vi "CalculateRotorBar.vi"(6 "Calculation Cache In":T2 {"speed initial conditions"."zoom FFT settings"."FFT settings"."window" items=["Rectangle"=0, "Hanning"=1, "Hamming"=2, "Blackman-Harris"=3, "Exact Blackman"=4, "Blackman"=5, "Flat Top"=6, "4 Term B-Harris "=7, "7 Term B-Harris"=8, "Low Sidelobe"=9, "Blackman Nuttall"=11, "Triangle"=30, "Bartlett-Hanning"=31, "Bohman"=32, "Parzen"=33, "Welch"=34, "Kaiser"=60, "Dolph-Chebyshev"=61, "Gaussian"=62]; "spectrum initial conditions"."zoom FFT settings"."FFT settings"."window" items=["Rectangle"=0, "Hanning"=1, "Hamming"=2, "Blackman-Harris"=3, "Exact Blackman"=4, "Blackman"=5, "Flat Top"=6, "4 Term B-Harris "=7, "7 Term B-Harris"=8, "Low Sidelobe"=9, "Blackman Nuttall"=11, "Triangle"=30, "Bartlett-Hanning"=31, "Bohman"=32, "Parzen"=33, "Welch"=34, "Kaiser"=60, "Dolph-Chebyshev"=61, "Gaussian"=62]}, 8 "error in (no error)":errorcluster, 9 "Map":T1, 10 "current waveform":waveform(dbl)[](array[waveform]), 11 "voltage waveform":waveform(dbl)[](array[waveform])) -> (0 "error out":errorcluster, 3 "max sideband magnitude [dB]":dbl, 4 "Calculation Cache Out":T2 {"speed initial conditions"."zoom FFT settings"."FFT settings"."window" items=["Rectangle"=0, "Hanning"=1, "Hamming"=2, "Blackman-Harris"=3, "Exact Blackman"=4, "Blackman"=5, "Flat Top"=6, "4 Term B-Harris "=7, "7 Term B-Harris"=8, "Low Sidelobe"=9, "Blackman Nuttall"=11, "Triangle"=30, "Bartlett-Hanning"=31, "Bohman"=32, "Parzen"=33, "Welch"=34, "Kaiser"=60, "Dolph-Chebyshev"=61, "Gaussian"=62]; "spectrum initial conditions"."zoom FFT settings"."FFT settings"."window" items=["Rectangle"=0, "Hanning"=1, "Hamming"=2, "Blackman-Harris"=3, "Exact Blackman"=4, "Blackman"=5, "Flat Top"=6, "4 Term B-Harris "=7, "7 Term B-Harris"=8, "Low Sidelobe"=9, "Blackman Nuttall"=11, "Triangle"=30, "Bartlett-Hanning"=31, "Bohman"=32, "Parzen"=33, "Welch"=34, "Kaiser"=60, "Dolph-Chebyshev"=61, "Gaussian"=62]})   [LabVIEW 2017, in "McsaAnalysisFunctions.lvlib"]
uses:
  <vilib>/addons/InsightCM/Utilities/Analysis/MCSA/McsaAnalysisFunctions.lvlib
  <vilib>/addons/InsightCM/Utilities/Analysis/MCSA/controls/McsaCalculationCache.ctl
  <vilib>/addons/Electrical Power/Motor Monitoring/subVIs/ep_Initial Conditions for MCSA Spectra.ctl
  <vilib>/addons/Electrical Power/Motor Monitoring/subVIs/ep_Demodulation Algorithm.ctl
  <vilib>/addons/Electrical Power/Motor Monitoring/subVIs/ep_Zoom FFT Settings.ctl
  <vilib>/addons/Electrical Power/Motor Monitoring/subVIs/ep_Initial Conditions for Speed Estimation.ctl
  <vilib>/addons/PointValueMap/controls/PointMap.ctl
  <vilib>/addons/Electrical Power/Motor Monitoring/subVIs/ep_Spectra Settings.ctl
  <vilib>/addons/Electrical Power/Motor Monitoring/MCSA Spectra (1 Motor with IC).vi
  <vilib>/addons/Electrical Power/Motor Monitoring/Broken Rotor Bar Harmonics (1 Motor).vi
  <vilib>/addons/Electrical Power/Motor Monitoring/NI_EP_Motor Monitoring.lvlib
  <vilib>/addons/PointValueMap/PointValueMap.lvlib
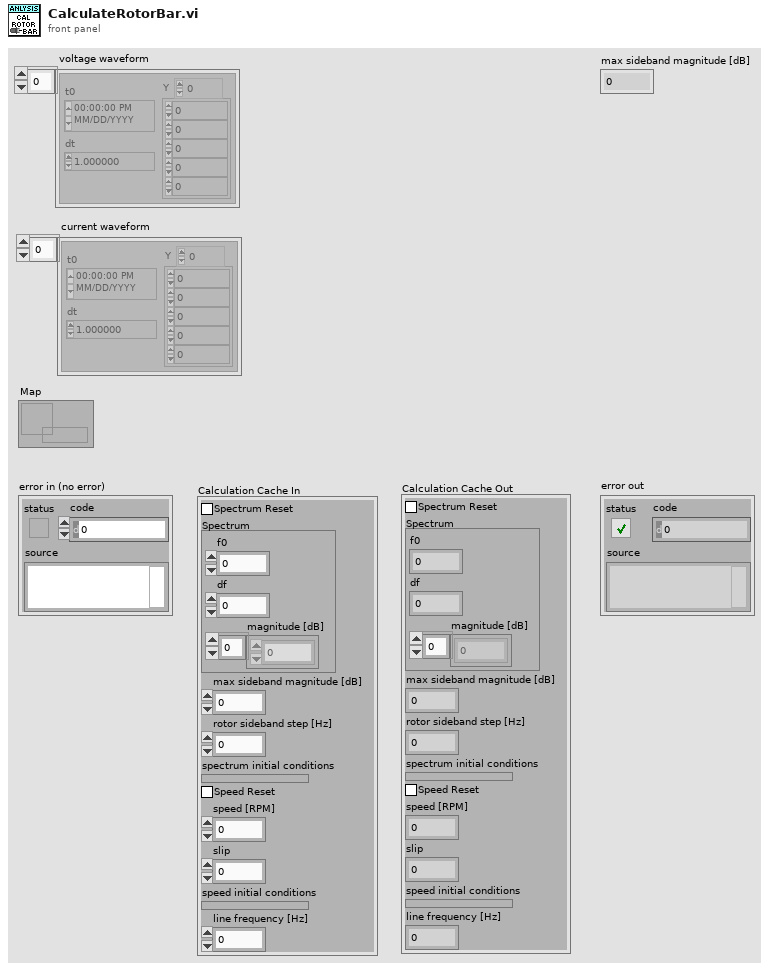
[diagram p1: front panel]
types:
  T1 = typedef "PointValueMap.lvlib/PointMap.ctl" = refnum<data-value>
  T2 = typedef "McsaAnalysisFunctions.lvlib/McsaCalculationCache.ctl" = cluster{"Spectrum Reset":bool, "Spectrum":cluster{"f0":dbl, "df":dbl, "magnitude [dB]":dbl[]}, "max sideband magnitude [dB]":dbl, "rotor sideband step [Hz]":dbl, "spectrum initial conditions":T3, "Speed Reset":bool, "speed [RPM]":dbl, "slip":dbl, "speed initial conditions":T6, "line frequency [Hz]":dbl}
  T3 = typedef "NI_EP_Motor Monitoring.lvlib/ep_Initial Conditions for MCSA Spectra.ctl" = cluster{"hilbert state":cluster{"delay conditions":dbl[], "filter conditions":dbl[]}, "zoom FFT state":cluster{"phase state":dbl, "zoom FFT state":cluster{"zoom settings state":cluster{"zoom":i32, "stop band attenuation":enum16{"84 dB", "96 dB", "120 dB"}, "alias protect in final transition":bool, "oversampling ratio":dbl}, "SML Decimation Filter (complex input) state":cluster{"decimation settings state":cluster{"M":i32, "stop band attenuation":enum16{"84 dB", "96 dB", "120 dB"}, "alias protect in transition band":bool, "oversampling ratio":dbl}, "counter for garbage samples state":i32, "sml_Parameter Setting for Zoom Factor state":cluster{"filter length * interpolation state":i32, "interpolation state":i32, "comb filter order state":i32, "CFIR par state":cluster{"h":dbl[], "M":i32, "N":i32}, "LFIR par state":cluster{"h":dbl[], "M":i32, "N":i32}, "CIC Stages state":i32}, "aal_CIC (complex input) state":cluster{"aal_cascaded moving average (complex input) state":cluster{"states":cdb[], "circular buffers state":cdb[][], "circular buffer counter state":i32}, "aal_moving average with decimation by order (complex input) state":cluster{"residue result state":cdb, "processed data counter state":i32}}, "sml_Cascaded Decimation Filter (complex input) CFIR state":cluster{"unprocessed data state":cdb[], "final conditions state":cdb[][], "sml_M-1 Decimator with IC (complex input) state":cluster{"coefficients in reverse order state":dbl[], "max index for coefficients state":i32}}, "sml_Cascaded Decimation Filter (complex input) LFIR state":cluster{"unprocessed data state":cdb[], "final conditions state":cdb[][], "sml_M-1 Decimator with IC (complex input) state":cluster{"coefficients in reverse order state":dbl[], "max index for coefficients state":i32}}}, "ma_SML Data Packing (complex input) state":cluster{"array getting packed state":cdb[], "last array processed state":cdb[], "index state":i32, "packing parameters state":cluster{i32, "size":i32}}}, "FFT{X} [Vrms]":cdb[]}, "IIR filter state":cluster{"filter state":dbl[]}, "demodulation settings":cluster{"enable? (F)":bool, "algorithm":T4}, "highpass IIR Filter":cluster{"filter structure":enum32{"IIR 2nd Order", "IIR 4th Order"}, "Reverse Coefficients":dbl[], "Forward Coefficients":dbl[]}, "Hilbert FIR filter":cluster{"coefficients":dbl[], "delay":i32}, "zoom FFT settings":T5}
  T4 = typedef "NI_EP_Motor Monitoring.lvlib/ep_Demodulation Algorithm.ctl" = enum16{"1-phase signal", "3-phase signals"}
  T5 = typedef "NI_EP_Motor Monitoring.lvlib/ep_Zoom FFT Settings.ctl" = cluster{"FFT settings":cluster{"window":u16, "Window Size":i32, "FFT Size":i32, "%overlap":dbl}, "zoom settings":cluster{"zoom":i32, "stop band attenuation":enum16{"84 dB", "96 dB", "120 dB"}, "alias protect in final transition":bool, "oversampling ratio":dbl}, "other settings":cluster{"fmod":dbl, "f0":dbl, "df":dbl, "oidx":i32, "olen":i32}, "iterations":i32, "max block size":i32, "fs":dbl}
  T6 = typedef "NI_EP_Motor Monitoring.lvlib/ep_Initial Conditions for Speed Estimation.ctl" = cluster{"SVAF state":cluster{"space vector amplitude":dbl, "hilbert state":cluster{"delay conditions":dbl[], "filter conditions":dbl[]}}, "zoom FFT state":cluster{"phase state":dbl, "zoom FFT state":cluster{"zoom settings state":cluster{"zoom":i32, "stop band attenuation":enum16{"84 dB", "96 dB", "120 dB"}, "alias protect in final transition":bool, "oversampling ratio":dbl}, "SML Decimation Filter (complex input) state":cluster{"decimation settings state":cluster{"M":i32, "stop band attenuation":enum16{"84 dB", "96 dB", "120 dB"}, "alias protect in transition band":bool, "oversampling ratio":dbl}, "counter for garbage samples state":i32, "sml_Parameter Setting for Zoom Factor state":cluster{"filter length * interpolation state":i32, "interpolation state":i32, "comb filter order state":i32, "CFIR par state":cluster{"h":dbl[], "M":i32, "N":i32}, "LFIR par state":cluster{"h":dbl[], "M":i32, "N":i32}, "CIC Stages state":i32}, "aal_CIC (complex input) state":cluster{"aal_cascaded moving average (complex input) state":cluster{"states":cdb[], "circular buffers state":cdb[][], "circular buffer counter state":i32}, "aal_moving average with decimation by order (complex input) state":cluster{"residue result state":cdb, "processed data counter state":i32}}, "sml_Cascaded Decimation Filter (complex input) CFIR state":cluster{"unprocessed data state":cdb[], "final conditions state":cdb[][], "sml_M-1 Decimator with IC (complex input) state":cluster{"coefficients in reverse order state":dbl[], "max index for coefficients state":i32}}, "sml_Cascaded Decimation Filter (complex input) LFIR state":cluster{"unprocessed data state":cdb[], "final conditions state":cdb[][], "sml_M-1 Decimator with IC (complex input) state":cluster{"coefficients in reverse order state":dbl[], "max index for coefficients state":i32}}}, "ma_SML Data Packing (complex input) state":cluster{"array getting packed state":cdb[], "last array processed state":cdb[], "index state":i32, "packing parameters state":cluster{i32, "size":i32}}}, "FFT{X} [Vrms]":cdb[]}, "speed state":cluster{"speed [RPM]":dbl, "slip":dbl}, "speed estimation settings":cluster{"% overlap":dbl, "algorithm":T4}, "filter information":cluster{"coefficients":dbl[], "order":i32}, "zoom FFT settings":T5, "last valid window":i32, "fund. frequency for averager":dbl[]}
  T7 = typedef "NI_EP_Motor Monitoring.lvlib/ep_Spectra Settings.ctl" = cluster{"number of lines":i32, "% overlap":dbl, "maximum frequency [Hz]":dbl}
  T8 = cluster{"f0":dbl, "df":dbl, "magnitude [dB]":dbl[]}
  T9 = cluster{"spectrum":cluster{"f0":dbl, "df":dbl, "magnitude [dB]":dbl[]}, "demodulated?":bool}
  T10 = cluster{"sideband frequency [Hz]":dbl[], "sideband magnitude [dB]":dbl[]}
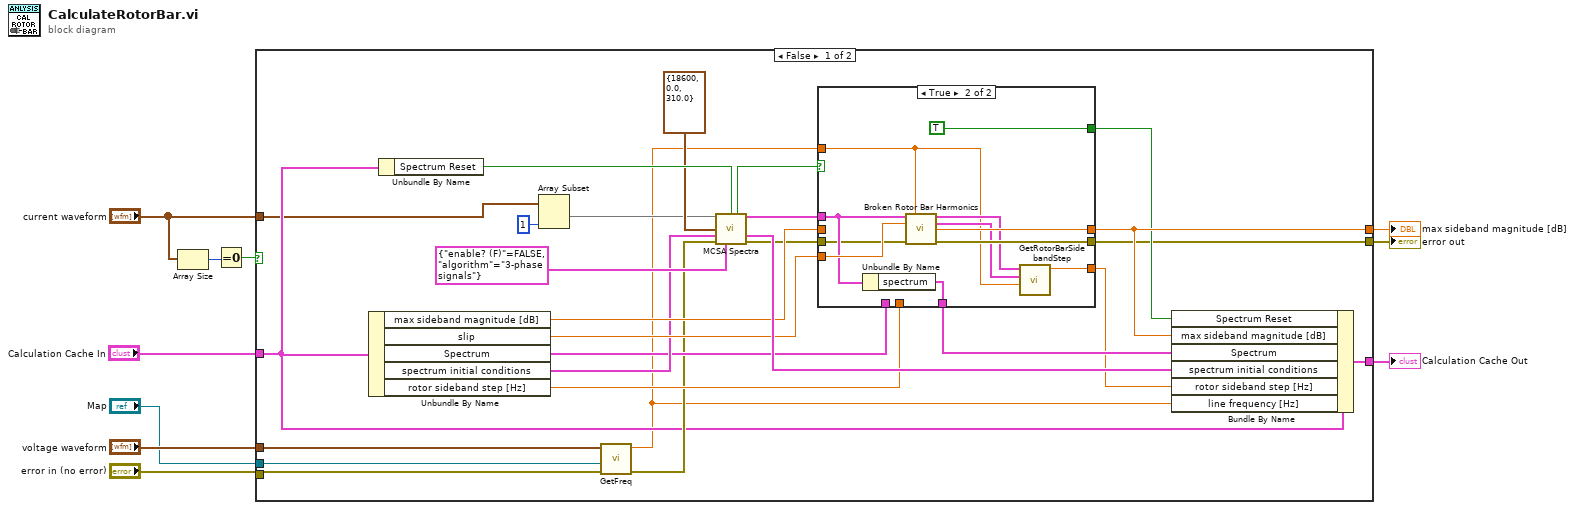
[diagram p0: block diagram]
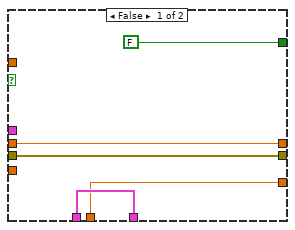
[diagram p2: hidden frame]
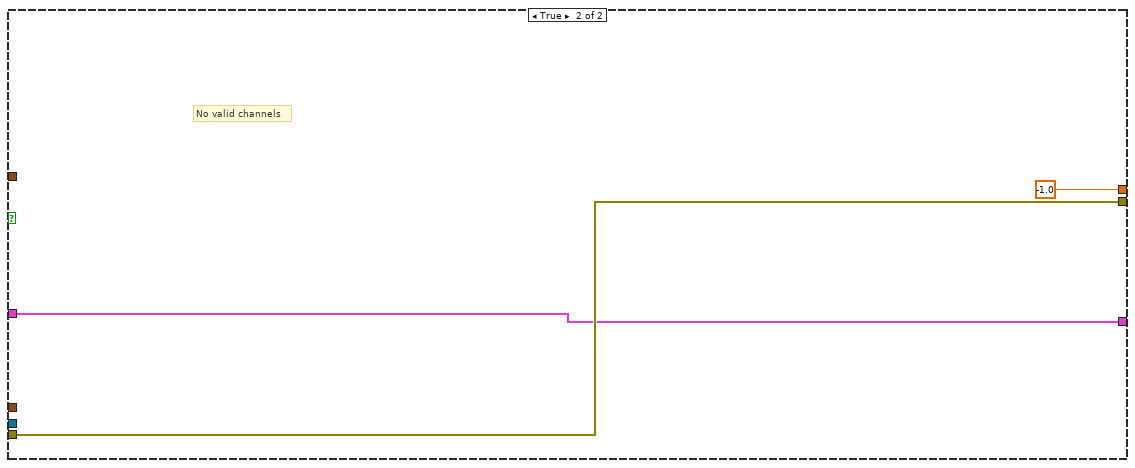
[diagram p3: hidden frame]
diagram:
  n1 = Array Size(array="current waveform") -> (size(s)=w1:i32)
  n2 = Equal To 0?(x=w1) -> (x = 0?=w2:bool)
  n3 = case shown="False" w2 {
    tunnel: "current waveform" -> [w13 _]
    tunnel: [w37 w54] -> w10
    tunnel: [w36 -1.0 ("max sideband magnitude [dB]")] -> w9
    tunnel: [w22 w55] -> w8
    tunnel: "error in (no error)" -> [w19 w55]
    tunnel: "Calculation Cache In" -> [w17 w54]
    tunnel: "voltage waveform" -> [w16 _]
    tunnel: "Map" -> [w15 _]
    frame False {
      n4 = Unbundle By Name(w17) -> ("max sideband magnitude [dB]"=w27:dbl, "slip"=w28:dbl, "Spectrum"=w25:T8, "spectrum initial conditions"=w26:T3, "rotor sideband step [Hz]"=w21:dbl)
      n5 = Unbundle By Name(w17) -> ("Spectrum Reset"=w35:bool)
      n6 = Array Subset(array=w13, length=1) -> (w14:waveform(dbl)[])  [unwired: 1 in]
      n7 = call <vilib>:"GetFreq.vi"("error in (no error)"=w19, "Map"=w15, "waveforms"=w16) -> ("error out"=w18:errorcluster, "frequency"=w11:dbl)  [unwired: 7 in]
      n8 = call-poly <vilib>:"MCSA Spectra.vi"("waveforms"=w14, "reset? (F)"=w35, "spectrum settings"=T7 {"number of lines"=18600, "% overlap"=0.0, "maximum frequency [Hz]"=310.0}, "initial conditions"=w26, "error in (no error)"=w18, "demodulation settings"=cluster{"enable? (F)":bool, "algorithm":T4} {"enable? (F)"=FALSE, "algorithm"=enum."3-phase signals"}) -> ("new spectrum available?"=w34:bool, "spectrum information"=w30:T9, "final conditions"=w31:T3, "error out"=w24:errorcluster)  [unwired: 6 in]
      n9 = case shown="True" w34 {
        tunnel: w11 -> [_ w43]
        tunnel: w30 -> [_ w50]
        tunnel: w28 -> [_ w53]
        tunnel: [FALSE ("Spectrum Reset") TRUE ("Spectrum Reset")] -> w29
        tunnel: [w41 w51] -> w36
        tunnel: w27 -> [w41 _]
        tunnel: [w40 w49] -> w23
        tunnel: w25 -> [w40 _]
        tunnel: w24 -> [w39 w48]
        tunnel: [w39 w47] -> w22
        tunnel: w21 -> [w38 _]
        tunnel: [w38 w45] -> w20
        frame False {
        }
        frame True {
          n10 = Unbundle By Name(w50) -> ("spectrum"=w49:T8)
          n11 = call-poly <vilib>:"Broken Rotor Bar Harmonics.vi"("spectrum information"=w50, "fundamental frequency [Hz]"=w43, "slip"=w53, "error in (no error)"=w48) -> ("upper sidebands"=w46:T10, "lower sidebands"=w44:T10, "max sideband magnitude [dB]"=w51:dbl, "error out"=w47:errorcluster)  [unwired: 8 in]
          n12 = call <vilib>:"GetRotorBarSidebandStep.vi"("line frequency [Hz]"=w43, "lower sidebands"=w44, "upper sidebands"=w46) -> ("Rotor Sideband Step [Hz]"=w45:dbl)  [unwired: 8 in]
        }
      }
      n13 = Bundle By Name(cluster=w17, "Spectrum Reset"=w29, "max sideband magnitude [dB]"=w36, "Spectrum"=w23, "spectrum initial conditions"=w31, "rotor sideband step [Hz]"=w20, "line frequency [Hz]"=w11) -> (w37:T2)
    }
    frame True {
      # "No valid channels"
    }
  }
  "max sideband magnitude [dB]" <- w9
  "Calculation Cache Out" <- w10
  "error out" <- w8
